vi "Write Setup.vi"(8 "error in":errorcluster, 10 "Setup Data":T1={"DataBase Data"={"Api Token"="", "Organization"="", "url"="", "Organization ID"=""}, "Write Data"={"Bucket"="", "Timestamp precision"=enum."Milliseconds", "Line protocol"="", "Measurement"=""}, "Query - csv"=""}, 11 "File Path":path) -> (0 "error out":errorcluster)   [LabVIEW 2020]
doc: "Writes all settings from the test application to the setup file"
uses:
  Setup Data.ctl
  Client/DataBase Data.ctl
  Client/Write Data.ctl
  Client/Write Precision.ctl
  <vilib>/Utility/xml.llb/Write to XML File(string).vi
  InfluxDB v2 Client.lvlib
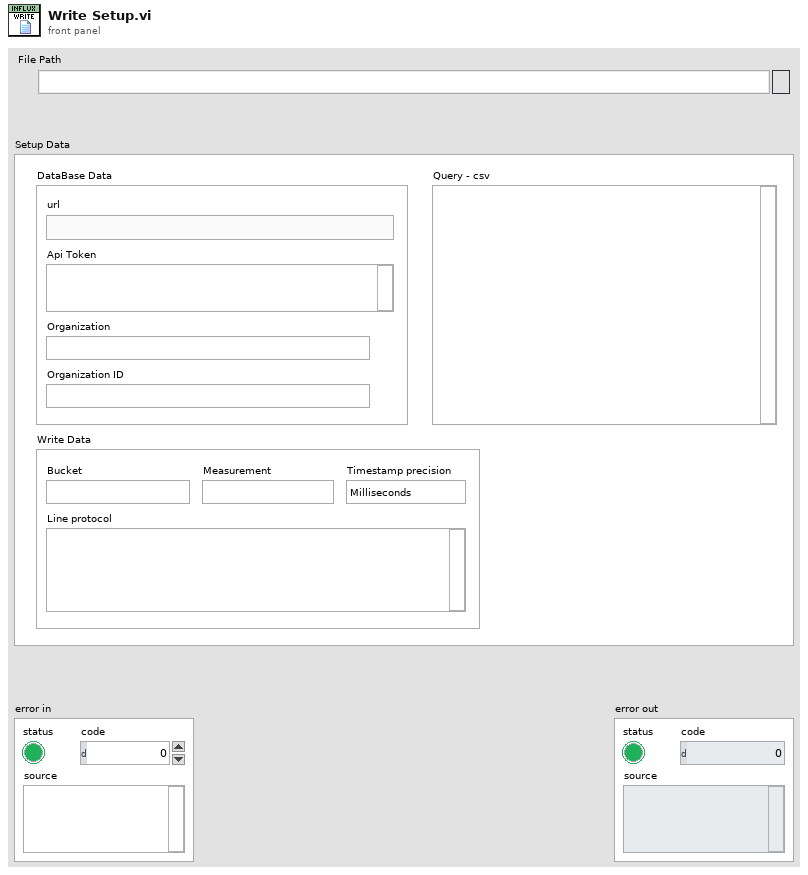
[diagram p1: front panel]
types:
  T1 = typedef "Setup Data.ctl" = cluster{"DataBase Data":T2, "Write Data":T3, "Query - csv":string}
  T2 = typedef "InfluxDB v2 Client.lvlib/DataBase Data.ctl" = cluster{"Api Token":string, "Organization":string, "url":string, "Organization ID":string}
  T3 = typedef "InfluxDB v2 Client.lvlib/Write Data.ctl" = cluster{"Bucket":string, "Timestamp precision":T4, "Line protocol":string, "Measurement":string}
  T4 = typedef "InfluxDB v2 Client.lvlib/Write Precision.ctl" = enum16{"Nanoseconds", "Microseconds", "Milliseconds", "Seconds"}
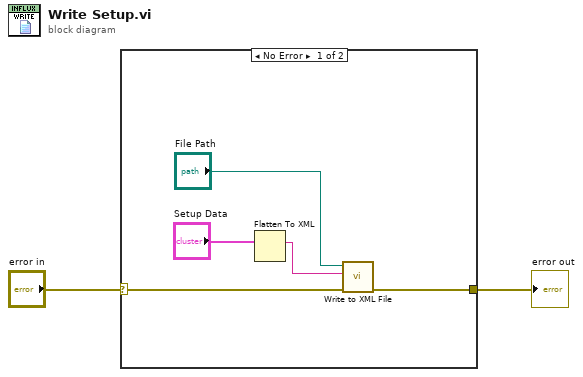
[diagram p0: block diagram]
diagram:
  n1 = case shown="No Error" "error in" {
    selector: "error in" -> [w6 w8]
    tunnel: [w3 w8] -> w1
    frame No Error {
      n2 = Flatten To XML(6:"Setup Data") -> (2:w5:string)
      n3 = call-poly <vilib>:"Write to XML File.vi"("error in (no error)"=w6, "XML Input"=w5, "XML File Path"="File Path") -> ("error out"=w3:errorcluster)  [unwired: 6 in, 2 out]
    }
    frame Error {
    }
  }
  "error out" <- w1
